vi "to string.vi"(8 "error in":errorcluster, 11 "byte":u8[](array[numeric]) format="%b") -> (0 "error out":errorcluster, 3 "String":string)   [LabVIEW 2020, in "MessagePack.lvlib" / "MessagePack.lvclass"]
uses:
  MessagePack.lvclass
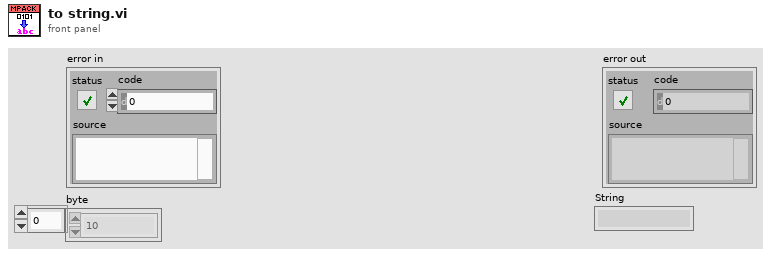
[diagram p1: front panel]
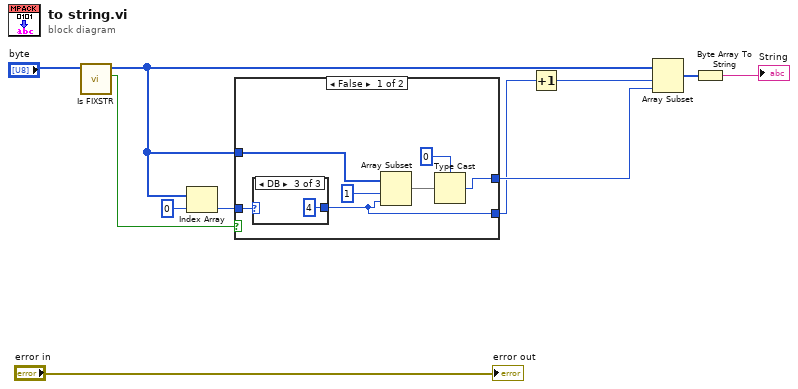
[diagram p0: block diagram]
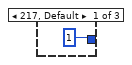
[diagram p2: hidden frame]
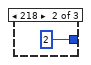
[diagram p3: hidden frame]
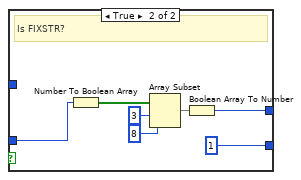
[diagram p4: hidden frame]
diagram:
  n1 = call "Is FIXSTR.vi"("bytes"="byte") -> ("Is FIXSTR?"=w10:bool, "bytes"=w6:u8[])  [unwired: 9 in]
  n2 = Index Array(array=w6, index=0) -> (element=w7:u8)
  n3 = case shown="False" w10 {
    tunnel: [w13 w25] -> w5
    tunnel: w7 -> [w18 w24]
    tunnel: [w12 1] -> w2
    tunnel: w6 -> [w17 _]
    frame False {
      n4 = case shown="DB" w18 {
        tunnel: [1 2 4] -> w12
        frame 217, Default {
        }
        frame 218 {
        }
        frame 219 {
        }
      }
      n5 = Array Subset(array=w17, index=1, length=w12) -> (w15:u8[])
      n6 = Type Cast(type=u32 0, x=w15) -> (*(type *) &x=w13:u32)
    }
    frame True {
      # "Is FIXSTR?"
      n7 = Number To Boolean Array(number=w24) -> (Boolean array=w23:bool[])
      n8 = Array Subset(array=w23, index=3, length=8) -> (w26:bool[])
      n9 = Boolean Array To Number(Boolean array=w26) -> (number=w25:u32)
    }
  }
  n10 = Increment(x=w2) -> (x+1=w1:i32)
  n11 = Array Subset(array=w6, index=w1, length=w5) -> (w4:u8[])
  n12 = Byte Array To String(unsigned byte array=w4) -> (string=→"String":string)
  "error out" <- "error in"
